vi "Launcher.vi"() -> ()   [LabVIEW 2021, in "Echo Broadcast with External Client.lvlib"]
uses:
  Echo Broadcast with External Client.lvlib
  WS Test Server/WS Test Server.lvclass
  C:/Program Files/National Instruments/LabVIEW 2021/vi.lib/ActorFramework/Actor/Actor.lvclass
  WebSocket Actor/WebSocket Server Manager/WebSocket Server Manager.lvclass
  WS Test Server/WS Test Server.lvclass/WS Test Server.ctl
  WS Test Server/properties/Write WebSocket Server Manager Enqueuer.vi
  <vilib>/ActorFramework/Actor/Actor.lvclass
panel:
  out "error out":errorcluster
  # "In this example the main actor allows the user to launch WebSocket Server Actors with user defined listener settings by means of the Server Manager Actor Infrastructure.  The user will then be able to add services to such server that will echo back the data sent by the client. You an use any client such as for example the one implemented as Chrome extension downloadable here \nhttps://chrome.google.com/webstore/detail/simple-websocket-client/pfdhoblngboilpfeibdedpjgfnlcodoo"
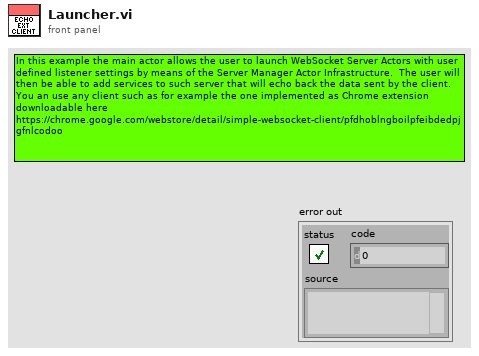
[diagram p1: front panel]
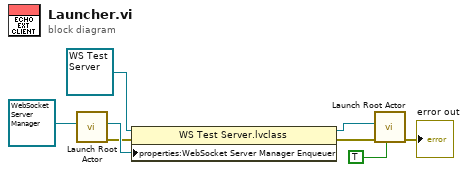
[diagram p0: block diagram]
diagram:
  n1 = call <vilib>:"Launch Root Actor.vi"("Actor"=refnum<class "WebSocket Server Manager.lvclass"> refnum ("WebSocket Actors.lvlib:WebSocket Server Manager.lvclass")) -> ("error out"=w2:errorcluster, "Actor's Enqueuer"=w3:refnum<class "Message Enqueuer.lvclass">)  [unwired: 9 in]
  n2 = property class="WS Test Server.lvclass"(reference=refnum<class "WS Test Server.lvclass"> refnum ("WS Full LabVIEW Test.lvlib:WS Test Server.lvclass"), error in=w2, "properties:WebSocket Server Manager Enqueuer"=w3) -> (reference out=w4:refnum<class "WS Test Server.lvclass">, error out=w1:errorcluster)
  n3 = call <vilib>:"Launch Root Actor.vi"("Open Actor Core front panel? (F)"=TRUE, "error in (no error)"=w1, "Actor"=w4) -> ("error out"=→"error out":errorcluster)  [unwired: 7 in, 1 out]
